vi "Counter1.vi"(6 "Action (Run)":T1=enum."Run", 8 "error in (no error)":errorcluster, 11 "Time To Elapse (2s)":dbl=2.0) -> (0 "error out":errorcluster, 1 "Time Elapsed?":bool, 3 "Time Elapsed [s]":dbl)   [LabVIEW 2020]
doc: "This VI checks if the Time To Elapse has Elapsed."
uses:
  #typedef_timer.ctl
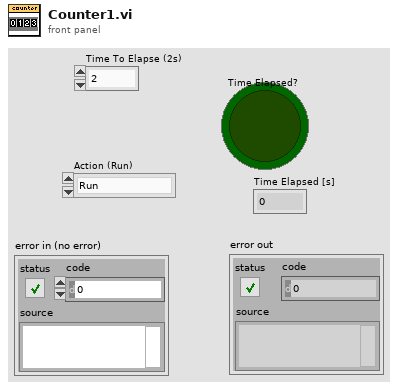
[diagram p1: front panel]
types:
  T1 = typedef "#typedef_timer.ctl" = enum16{"Reset", "Run"}
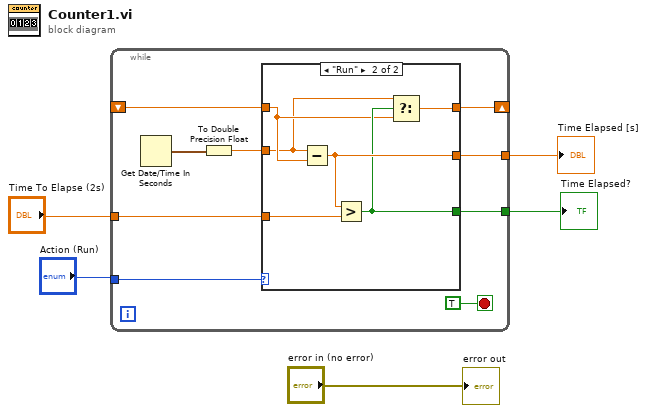
[diagram p0: block diagram]
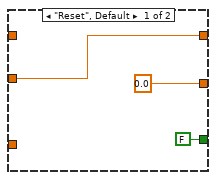
[diagram p2: hidden frame]
diagram:
  n1 = while {
    shift-right: [w9] -> _
    shift-left: _ -> [w10]
    tunnel: "Action (Run)" -> [w6]
    tunnel: [w13] -> w5
    tunnel: "Time To Elapse (2s)" -> [w8]
    tunnel: [w7] -> w1
    stop <- TRUE stop-if-true
    n2 = Get Date/Time In Seconds() -> (seconds since 1Jan1904=w12:timestamp)
    n3 = To Double Precision Float(number=w12) -> (double precision float=w11:dbl)
    n4 = case shown="\"Run\"" w6 {
      tunnel: w11 -> [w16 w18]
      tunnel: w10 -> [_ w20]
      tunnel: [w16 w19] -> w9
      tunnel: [0.0 w22] -> w13
      tunnel: w8 -> [_ w23]
      tunnel: [FALSE w21] -> w7
      frame "Reset", Default {
      }
      frame "Run" {
        n5 = Subtract(x=w18, y=w20) -> (x-y=w22:dbl)
        n6 = Greater?(x=w22, y=w23) -> (0:w21:bool)
        n7 = Select(t=w18, s=w21, f=w20) -> (s? t:f=w19:dbl)
      }
    }
  }
  "Time Elapsed [s]" <- w5
  "Time Elapsed?" <- w1
  "error out" <- "error in (no error)"
